vi "PH_Tektronix_7000.ProcEvents.vi"(0 "i ref in":refnum<vi>, 5 "error in":errorcluster) -> (14 "i ref out":refnum<vi>, 19 "error out":errorcluster)   [LabVIEW 2014, in "PH_Tektronix_7000.lvlib"]
doc: "This method is used to define the events the object will listen to. Add your own events here."
uses:
  PH_Tektronix_7000.lvlib
  CSCore/BaseProcess/BaseProcess.event definition.ctl
  CSCore/CAEObj/CAEObj.event definition.ctl
  CSCore/BaseProcess/BaseProcess.descriptor string definition.ctl
  CSCore/BaseProcess/BaseProcess.lvlib
  CSCore/CAEObj/CAEObj.lvlib
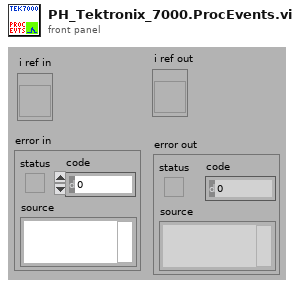
[diagram p1: front panel]
types:
  T1 = typedef "BaseProcess.lvlib/BaseProcess.event definition.ctl" = cluster{"CAEEvtDef":T2, "Data Descriptor":T3}
  T2 = typedef "CAEObj.lvlib/CAEObj.event definition.ctl" = cluster{"URL":string, "enable":bool, "ignoreResID":bool}
  T3 = typedef "BaseProcess.lvlib/BaseProcess.descriptor string definition.ctl" = string
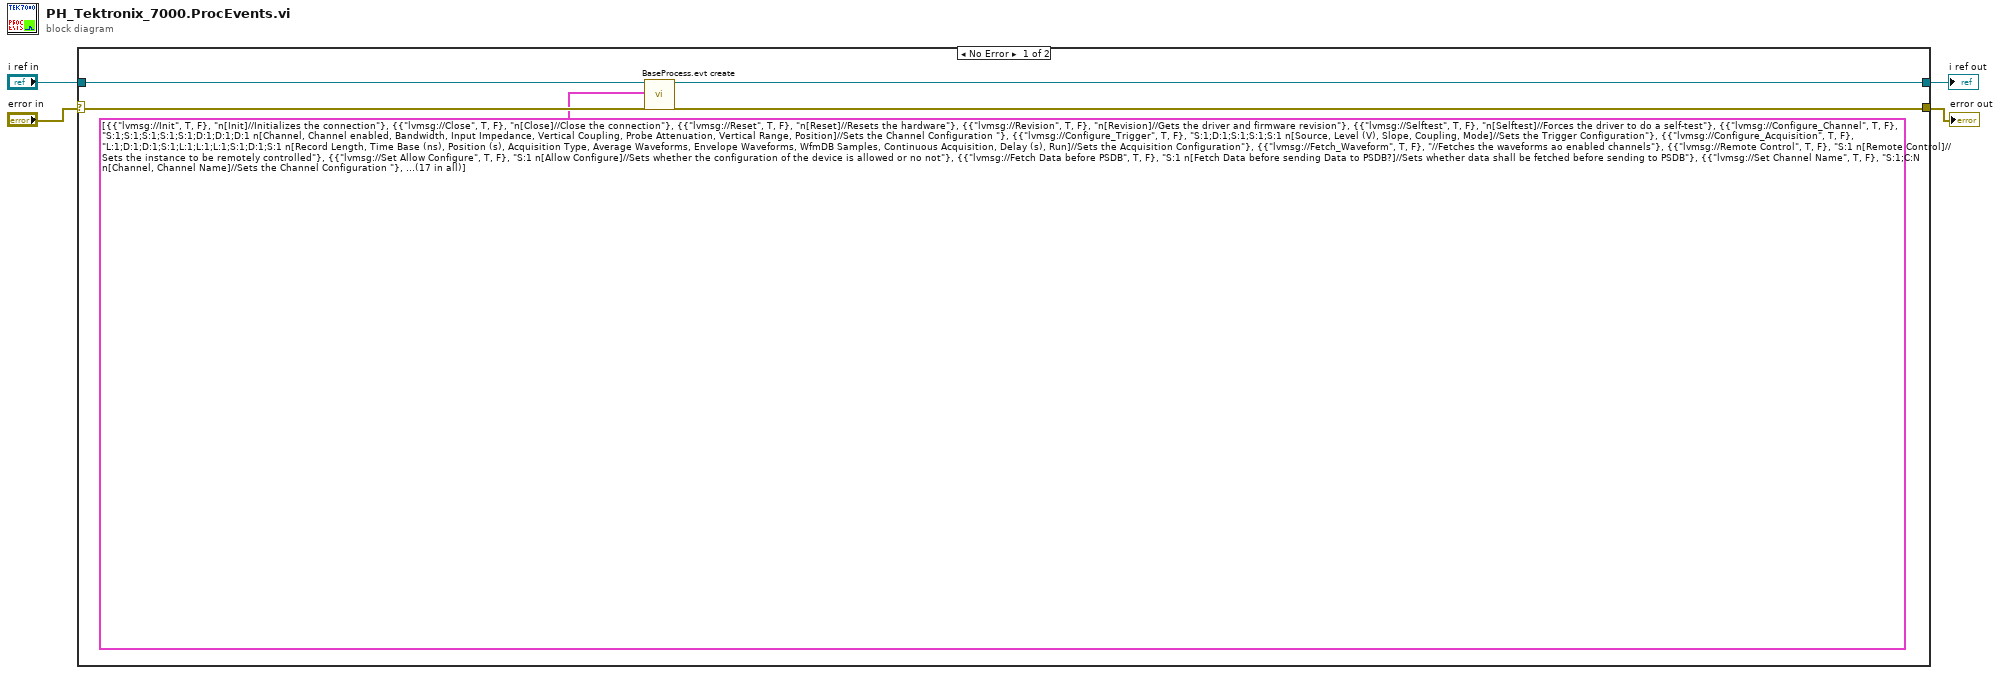
[diagram p0: block diagram]
diagram:
  n1 = case shown="No Error" "error in" {
    selector: "error in" -> [w7 w10]
    tunnel: "i ref in" -> [w6 w11]
    tunnel: [w9 w11] -> w3
    tunnel: [w8 w10] -> w2
    frame No Error {
      n2 = call "BaseProcess.evt create.vi"("i ref in"=w6, "newEvents"=T1[] [{"CAEEvtDef"={"URL"="lvmsg://Init", "enable"=TRUE, "ignoreResID"=FALSE}, "Data Descriptor"="n[Init]//Initializes the connection"}, {"CAEEvtDef"={"URL"="lvmsg://Close", "enable"=TRUE, "ignoreResID"=FALSE}, "Data Descriptor"="n[Close]//Close the connection"}, {"CAEEvtDef"={"URL"="lvmsg://Reset", "enable"=TRUE, "ignoreResID"=FALSE}, "Data Descriptor"="n[Reset]//Resets the hardware"}, {"CAEEvtDef"={"URL"="lvmsg://Revision", "enable"=TRUE, "ignoreResID"=FALSE}, "Data Descriptor"="n[Revision]//Gets the driver and firmware revision"}, {"CAEEvtDef"={"URL"="lvmsg://Selftest", "enable"=TRUE, "ignoreResID"=FALSE}, "Data Descriptor"="n[Selftest]//Forces the driver to do a self-test"}, {"CAEEvtDef"={"URL"="lvmsg://Configure_Channel", "enable"=TRUE, "ignoreResID"=FALSE}, "Data Descriptor"="S:1;S:1;S:1;S:1;S:1;D:1;D:1;D:1 n[Channel, Channel enabled, Bandwidth, Input Impedance, Vertical Coupling, Probe Attenuation, Vertical Range, Position]//Sets the Channel Configuration "}, {"CAEEvtDef"={"URL"="lvmsg://Configure_Trigger", "enable"=TRUE, "ignoreResID"=FALSE}, "Data Descriptor"="S:1;D:1;S:1;S:1;S:1 n[Source, Level (V), Slope, Coupling, Mode]//Sets the Trigger Configuration"}, {"CAEEvtDef"={"URL"="lvmsg://Configure_Acquisition", "enable"=TRUE, "ignoreResID"=FALSE}, "Data Descriptor"="L:1;D:1;D:1;S:1;L:1;L:1;L:1;S:1;D:1;S:1 n[Record Length, Time Base (ns), Position (s), Acquisition Type, Average Waveforms, Envelope Waveforms, WfmDB Samples, Continuous Acquisition, Delay (s), Run]//Sets the Acquisition Configuration"}, {"CAEEvtDef"={"URL"="lvmsg://Fetch_Waveform", "enable"=TRUE, "ignoreResID"=FALSE}, "Data Descriptor"="//Fetches the waveforms ao enabled channels"}, {"CAEEvtDef"={"URL"="lvmsg://Remote Control", "enable"=TRUE, "ignoreResID"=FALSE}, "Data Descriptor"="S:1 n[Remote Control]//Sets the instance to be remotely controlled"}, {"CAEEvtDef"={"URL"="lvmsg://Set Allow Configure", "enable"=TRUE, "ignoreResID"=FALSE}, "Data Descriptor"="S:1 n[Allow Configure]//Sets whether the configuration of the device is allowed or no not"}, {"CAEEvtDef"={"URL"="lvmsg://Fetch Data before PSDB", "enable"=TRUE, "ignoreResID"=FALSE}, "Data Descriptor"="S:1 n[Fetch Data before sending Data to PSDB?]//Sets whether data shall be fetched before sending to PSDB"}, {"CAEEvtDef"={"URL"="lvmsg://Set Channel Name", "enable"=TRUE, "ignoreResID"=FALSE}, "Data Descriptor"="S:1;C:N n[Channel, Channel Name]//Sets the Channel Configuration "}, {"CAEEvtDef"={"URL"="lvmsg://get Channel Config", "enable"=TRUE, "ignoreResID"=FALSE}, "Data Descriptor"="S:1 n[Channel]//Querries the hardware for the Channel configuration"}, {"CAEEvtDef"={"URL"="lvmsg://get Acquisition Config", "enable"=TRUE, "ignoreResID"=FALSE}, "Data Descriptor"="//Querries the hardware for the Acquisition configuration"}, {"CAEEvtDef"={"URL"="lvmsg://get Trigger Config", "enable"=TRUE, "ignoreResID"=FALSE}, "Data Descriptor"="//Querries the hardware for the Trigger configuration"}, {"CAEEvtDef"={"URL"="lvmsg://SetPeriodicInterval", "enable"=TRUE, "ignoreResID"=FALSE}, "Data Descriptor"="L:1 n[Periodic Interval (ms)// Sets the periodic interval in milliseconds"}] ("new events"), "error in (no error)"=w7) -> ("i ref out"=w9:refnum<vi>, "error out"=w8:errorcluster)  [unwired: 13 in, 2 out]
    }
    frame Error {
    }
  }
  "i ref out" <- w3
  "error out" <- w2
